vi "Write AirMass.vi"(8 "error in (no error)":errorcluster, 10 "AirMass":string, 11 "TCS in":refnum<class "TCS.lvclass">) -> (0 "error out":errorcluster, 3 "TCS out":refnum<class "TCS.lvclass">)   [LabVIEW 2018, in "TCS.lvclass"]
uses:
  TCS.lvclass
  TCS.lvclass/TCS.ctl
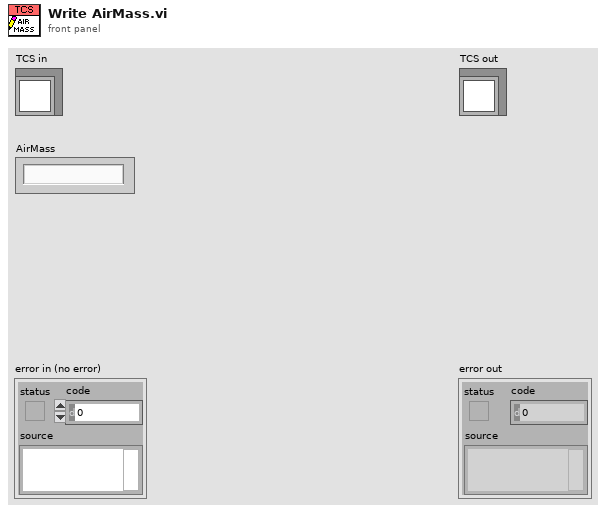
[diagram p1: front panel]
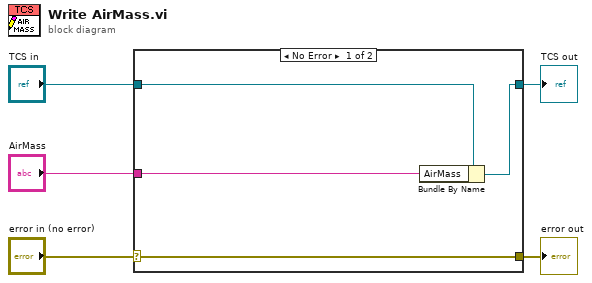
[diagram p0: block diagram]
diagram:
  n1 = case shown="No Error" "error in (no error)" {
    selector: "error in (no error)" -> [w9 w10]
    tunnel: [w9 w10] -> w4
    tunnel: [w7 w11] -> w2
    tunnel: "TCS in" -> [w8 w11]
    tunnel: "AirMass" -> [w6 _]
    frame No Error {
      n2 = Bundle By Name(cluster=w8, "AirMass"=w6) -> (w7:refnum<class "TCS.lvclass">)
    }
    frame Error {
    }
  }
  "error out" <- w4
  "TCS out" <- w2
